vi "table column sketch.vi"() -> ()   [LabVIEW 2020]
uses:
  source/Database OOP/Table/Table Class/Table.lvclass
  source/Database OOP/ADODB/ADODB Class/ADODB.lvclass
  C:/Users/User/Desktop/Raman Program/Database OOP/source/Database OOP/Database Interfaces/Database Advanced Schema Class/Database Adv Schema.lvclass
  source/Database OOP/ADODB/UDL Connection Class/UDL Connection.lvclass
  C:/Users/User/Desktop/Raman Program/Database OOP/source/Database OOP/Database Interfaces/Database Connection Class/Database Connection.lvclass
  source/Database OOP/Table Configuration Adv Schema DB/Table Configuration Adv Schema DB.lvclass
  C:/Users/User/Desktop/Raman Program/Database OOP/source/Database OOP/Table Configuration Interface/Table Configuration Interface.lvclass
  source/Database OOP/Table Configuration Adv Schema DB/Table Constructor Adv Schema DB.vi
  source/Database OOP/Database Interfaces/Database Interface Class/Database Interface.lvclass
  source/Database OOP/Table.lvlib
  C:/Users/User/Desktop/Raman Program/Database OOP/source/Database OOP/Database Interfaces/Database Interface Class/Database Interface.lvclass
  C:/Users/User/Desktop/Raman Program/Database OOP/source/Database OOP/ADODB/ADODB Class/ADODB.lvclass
panel:
  out "Table Control":string[][](table)
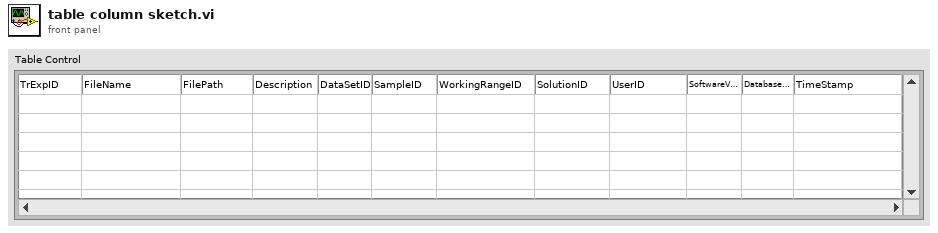
[diagram p1: front panel]
types:
  T1 = cluster{"Description":string, "SampleID":i32, "TimeStamp":timestamp}
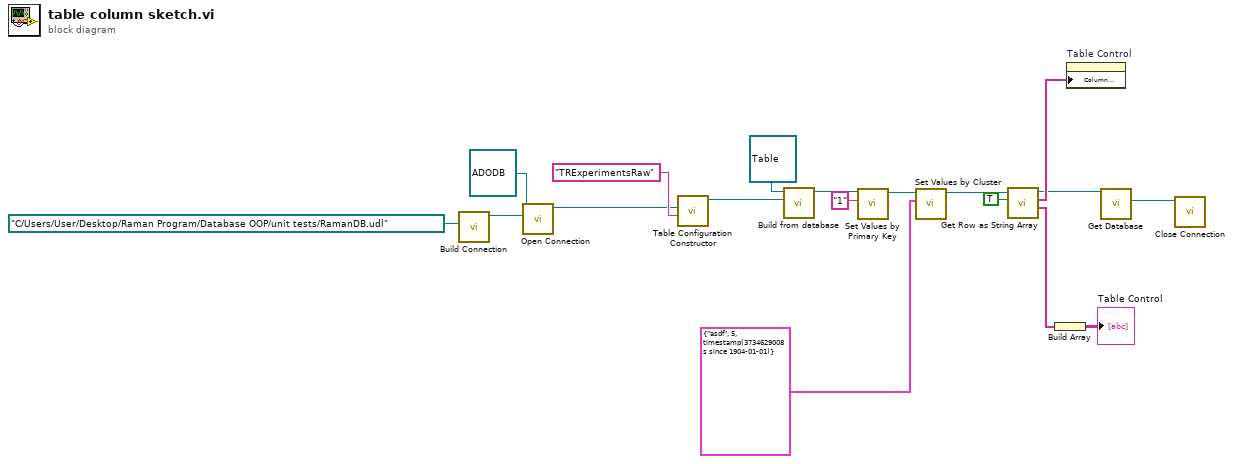
[diagram p0: block diagram]
diagram:
  n1 = call "Build Connection.vi"("*.udl file path"=path "C:/Users/User/Desktop/Raman Program/Database OOP/unit tests/RamanDB.udl") -> ("UDL Connection out"=w16:refnum<class "UDL Connection.lvclass">)  [unwired: 9 in, 1 out]
  n2 = call-dynamic "Open Connection.vi"("Connection"=w16, "ADODB in"=refnum<class "ADODB.lvclass"> refnum) -> ("ADODB out"=w13:refnum<class "ADODB.lvclass">)  [unwired: 8 in, 1 out]
  n3 = call-poly "Table Configuration Constructor.vi"("Table Name"="TRExperimentsRaw", "Database"=w13) -> ("Table Configuration Adv Schema DB out"=w18:refnum<class "Table Configuration Adv Schema DB.lvclass">)  [unwired: 8 in, 1 out]
  n4 = call-dynamic "Build from database.vi"("Table Configuration"=w18, "Table in"=refnum<class "Table.lvclass"> refnum ("Table.lvlib:Table.lvclass")) -> ("Table out"=w6:refnum<class "Table.lvclass">)  [unwired: 8 in, 1 out]
  n5 = call "Set Values by Primary Key.vi"("Primary Key Value"="1", "Table in"=w6) -> ("Table out"=w2:refnum<class "Table.lvclass">)  [unwired: 8 in, 1 out]
  n6 = call "Set Values by Cluster.vi"("Cluster"=T1 {"Description"="asdf", "SampleID"=5, "TimeStamp"=timestamp(3734629008.669306 s since 1904-01-01)}, "Table in"=w2) -> ("Table out"=w1:refnum<class "Table.lvclass">)  [unwired: 8 in, 1 out]
  n7 = call "Get Row as String Array.vi"("Preserve DB Column Order (F)"=TRUE, "Table in"=w1) -> ("Row Values"=w10:string[], "Column Names"=w8:string[], "Table out"=w7:refnum<class "Table.lvclass">)  [unwired: 6 in, 1 out]
  n8 = Build Array(w10) -> (→"Table Control":string[][])
  n9 = property on="Table Control" class="Tbl (strict)"("Column Headers[]"=w8) -> ()  [unwired: 2 in, 2 out]
  n10 = call "Get Database.vi"("Table in"=w7) -> ("Database Out"=w11:refnum<class "Database Interface.lvclass">)  [unwired: 8 in, 2 out]
  n11 = call-dynamic "Close Connection.vi"("Database Interface in"=w11) -> ()  [unwired: 9 in, 2 out]
